vi "AMI1700eth_init.vi"(8 "error in":errorcluster, 10 "port":u16, 11 "address":string) -> (0 "error out":errorcluster, 3 "conn_id":refnum<k5>, 4 "status":bool)   [LabVIEW 2019]
panel:
  out "string":string
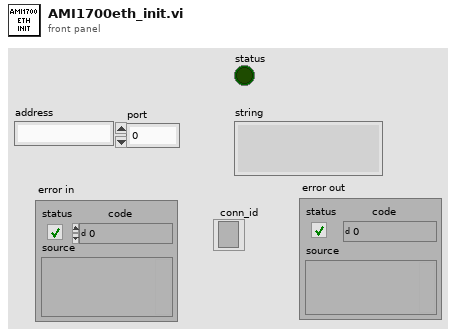
[diagram p1: front panel]
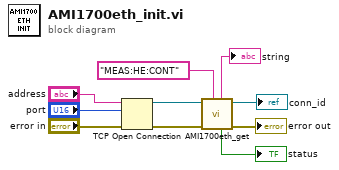
[diagram p0: block diagram]
diagram:
  n1 = TCP Open Connection(address="address", remote port or service name="port", error in (no error)="error in") -> (connection ID=w6:refnum<k5>, error out=w7:errorcluster)  [unwired: 2 in]
  n2 = call "AMI1700eth_get.vi"("command"="MEAS:HE:CONT", "error in"=w7, "conn_id_in"=w6) -> ("error out"=→"error out":errorcluster, "conn_id_out"=→"conn_id":refnum<k5>, "status"=→"status":bool, "string"=→"string":string)  [unwired: 5 in]
